vi "CAM_ATTEMPT_complex.vi"() -> ()   [LabVIEW 2021]
uses:
  C:/Program Files/Thorlabs/Scientific Imaging/DCx Camera Support/Develop/DotNet/uc480DotNet.dll
  Program Files/Thorlabs/Scientific Imaging/DCx Camera Support/Develop/DotNet/uc480DotNet.dll
panel:
  out "Camera ID":i32
  in  "String 2":string="C:\\Users\\marsan18\\Desktop\\Trial\\"
  out "Number of loops":i32
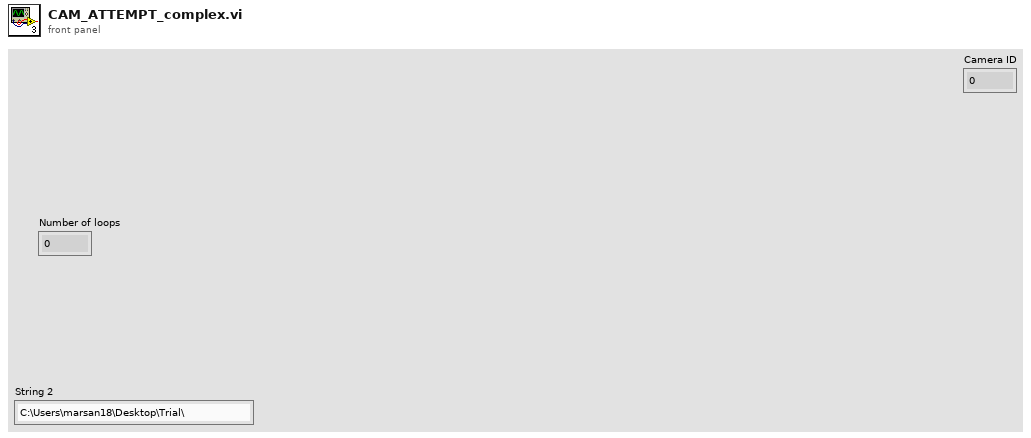
[diagram p1: front panel]
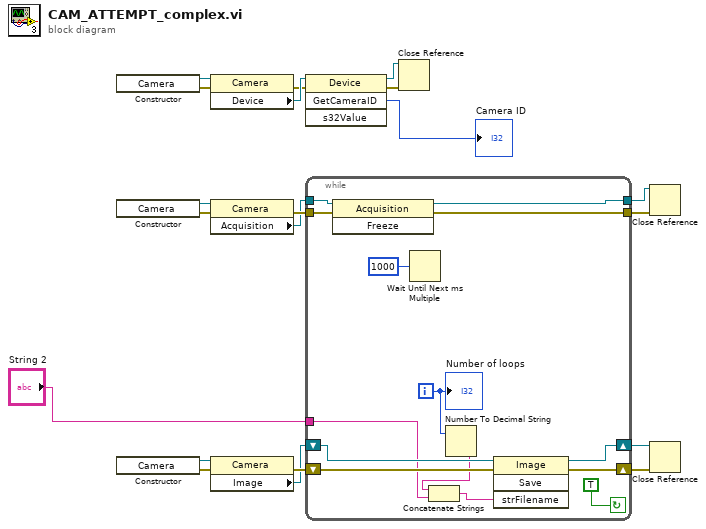
[diagram p0: block diagram]
diagram:
  n1 = constructor class="Camera"() -> (reference out=w7:refnum<k24>, error out=w8:errorcluster)  [unwired: 3 in, 1 out]
  n2 = constructor class="Camera"() -> (reference out=w13:refnum<k24>, error out=w14:errorcluster)  [unwired: 3 in, 1 out]
  n3 = constructor class="Camera"() -> (reference out=w17:refnum<k24>, error out=w18:errorcluster)  [unwired: 3 in, 1 out]
  n4 = property class="Camera"(reference=w7, error in=w8) -> (error out=w5:errorcluster, "Device"=w6:refnum<k24>)  [unwired: 1 out]
  n5 = property class="Camera"(reference=w13, error in=w14) -> (error out=w10:errorcluster, "Acquisition"=w9:refnum<k24>)  [unwired: 1 out]
  n6 = property class="Camera"(reference=w17, error in=w18) -> (error out=w20:errorcluster, "Image"=w19:refnum<k24>)  [unwired: 1 out]
  n7 = invoke class="Device" method="GetCameraID"(reference=w6, error in=w5) -> (reference out=w4:refnum<k24>, error out=w3:errorcluster, "GetCameraID"=→"Camera ID":i32)  [unwired: 2 in, 1 out]
  n8 = while {
    shift-right: [w31] -> w15
    shift-left: w20 -> [w34]
    shift-right: [w32] -> w16
    shift-left: w19 -> [w33]
    tunnel: [w28] -> w12
    tunnel: [w27] -> w11
    tunnel: w10 -> [w26]
    tunnel: w9 -> [w25]
    tunnel: "String 2" -> [w21]
    i -> [w24]
    stop <- TRUE continue-if-true
    n9 = invoke class="Acquisition" method="Freeze"(reference=w25, error in=w26) -> (reference out=w28:refnum<k24>, error out=w27:errorcluster)  [unwired: 1 in, 1 out]
    n10 = Wait Until Next ms Multiple(millisecond multiple=1000) -> ()  [unwired: 1 out]
    n11 = Number To Decimal String(number=w24) -> (decimal integer string=w23:string)  [unwired: 1 in]
    n12 = Concatenate Strings(w23, w21) -> (w22:string)
    n13 = invoke class="Image" method="Save"(reference=w33, error in=w34, "strFilename"=w22) -> (reference out=w32:refnum<k24>, error out=w31:errorcluster)  [unwired: 1 in, 2 out]
    "Number of loops" <- w24
  }
  n14 = Close Reference(reference=w4, error in (no error)=w3) -> ()  [unwired: 1 out]
  n15 = Close Reference(reference=w12, error in (no error)=w11) -> ()  [unwired: 1 out]
  n16 = Close Reference(reference=w16, error in (no error)=w15) -> ()  [unwired: 1 out]
